vi "Flow Observed Starts.vi"(2 "Reset Starts":bool, 7 "Flows":fxp<+/-,28,17>[](array[numeric])=[0.0, 0.0, 0.0, 0.0, 0.0, 0.0]) -> (8 "Observed Starts":u32[](array[numeric]))   [LabVIEW 2019]
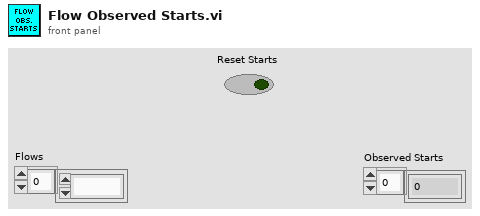
[diagram p1: front panel]
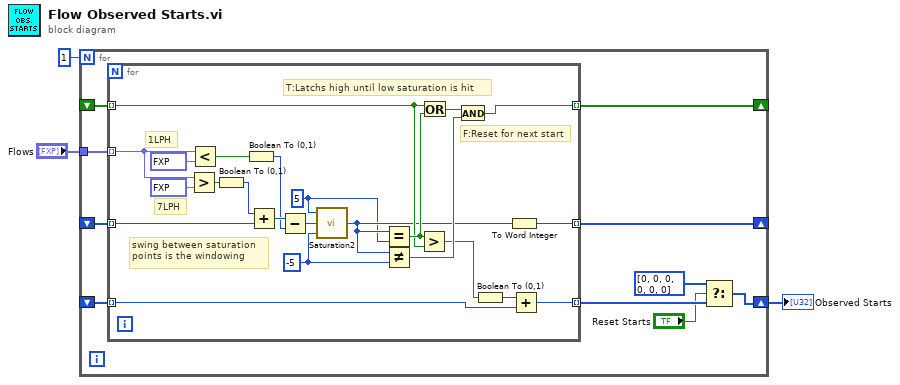
[diagram p0: block diagram]
diagram:
  n1 = for {
    N: 1 -> [_]
    tunnel: "Flows" -> [w13]
    shift-right: [w12] -> _
    shift-left: _ -> [w11]
    shift-right: [w10] -> _
    shift-left: _ -> [w9]
    shift-right: [w6] -> w2
    shift-left: _ -> [w8]
    n2 = for {
      tunnel: w13 -> [w25] mode=indexing
      tunnel: w11 -> [w24] mode=indexing
      tunnel: [w23] -> w12 mode=indexing
      tunnel: [w20] -> w10 mode=indexing
      tunnel: w9 -> [w22] mode=indexing
      tunnel: w8 -> [w14] mode=indexing
      tunnel: [w17] -> w7 mode=indexing
      w15 = -5 ("y")
      w16 = 5 ("y")
      # "T:Latchs high until low saturation is hit"
      # "swing between saturation\npoints is the windowing"
      # "F:Reset for next start"
      # "1LPH"
      # "7LPH"
      n3 = Greater?(x=w25, y=fxp<+/-,28,17> 13719.0) -> (0:w31:bool)
      n4 = Less?(x=w25, y=fxp<+/-,28,17> 13194.0) -> (x < y?=w32:bool)
      n5 = Boolean To (0,1)(Boolean=w31) -> (0, 1=w27:i16)
      n6 = Boolean To (0,1)(Boolean=w32) -> (0, 1=w26:i16)
      n7 = Add(x=w27, y=w22) -> (x+y=w34:i16)
      n8 = Subtract(x=w34, y=w26) -> (x-y=w33:i16)
      n9 = call "Saturation2"("upper limit"=w16, "input"=w33, "lower limit"=w15) -> ("output"=w21:i32)  [unwired: 6 in]
      n10 = Equal?(x=w21, y=w16) -> (x = y?=w30:bool)
      n11 = Not Equal?(x=w21, y=w15) -> (x != y?=w28:bool)
      n12 = Greater?(x=w30, y=w24) -> (0:w19:bool)
      n13 = Or(x=w24, y=w30) -> (x .or. y?=w29:bool)
      n14 = And(x=w29, y=w28) -> (x .and. y?=w23:bool)
      n15 = Boolean To (0,1)(Boolean=w19) -> (0, 1=w18:i16)
      n16 = To Word Integer(number=w21) -> (16bit integer=w20:i16)
      n17 = Add(x=w18, y=w14) -> (x+y=w17:u32)
    }
    n18 = Select(t=u32[] [0, 0, 0, 0, 0, 0], s="Reset Starts", f=w7) -> (s? t:f=w6:u32[])
  }
  "Observed Starts" <- w2
